vi "Autonomous.vi"   [LabVIEW 2019]
doc: "This VI starts when autonomous period begins, and will automatically be terminated when it ends. You can carry out timed or sensor driven operations directly to I/O or to subsystems without needing to return to the caller."
uses:
  <vilib>/Rock Robotics/WPI/Solenoid/WPI_SolenoidValue.ctl
  <vilib>/Rock Robotics/Network Tables/NT Read String.vi
  Framework/Robot Global Data.vi
types:
  T1 = typedef "WPI_SolenoidValue.ctl" = enum16{"Off", "On", "Forward", "Reverse"}
  T2 = typedef "Command Status Info.ctl" = cluster{"Name":string, "Status":T3, "notifier out":T4}
  T3 = typedef "Completion Status.ctl" = enum16{"Successful", "Aborted", "Incomplete"}
  T4 = typedef "Completion Notifier.ctl" = refnum<notifier>
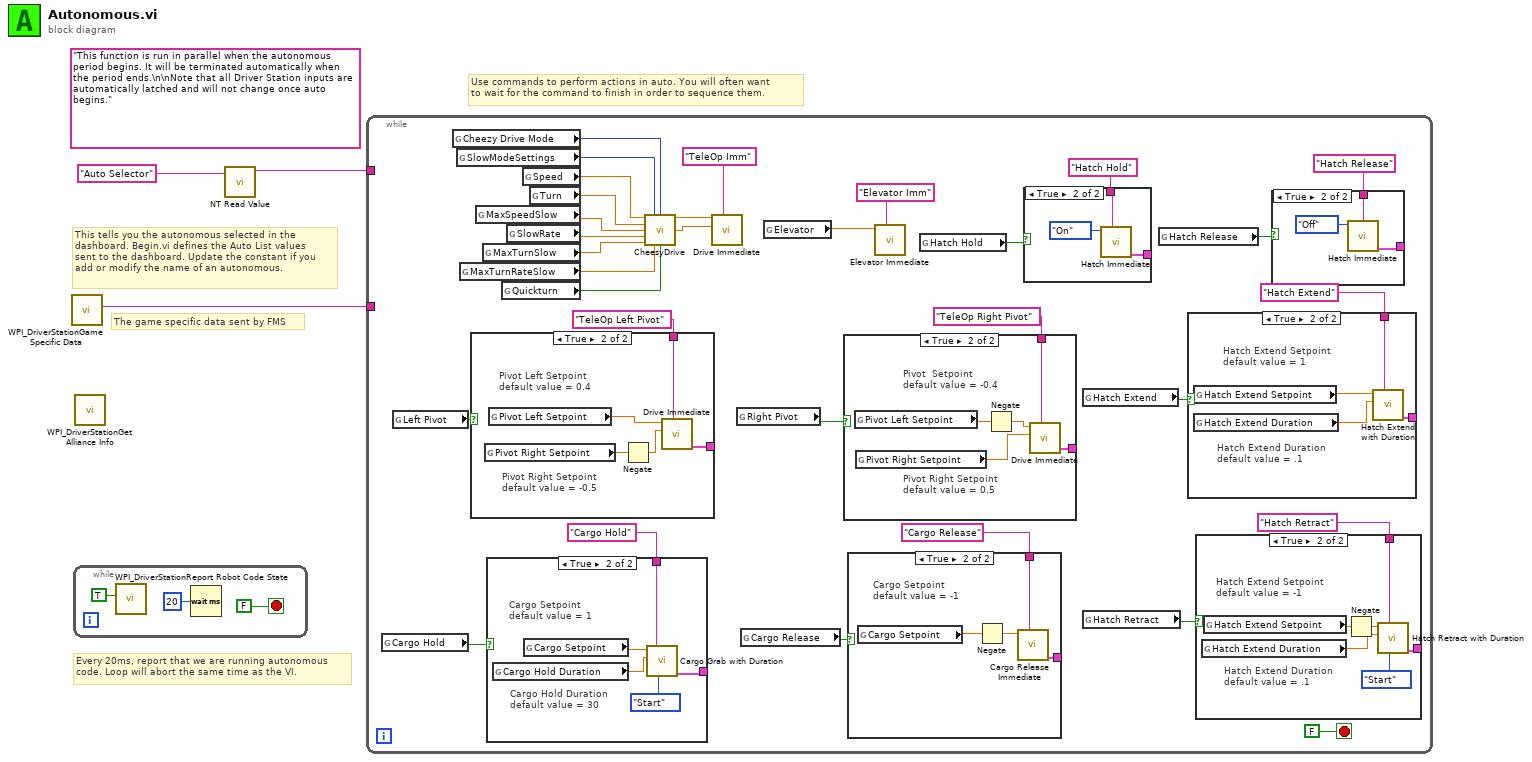
[diagram p0: block diagram]
diagram:
  (unwired) "This function is run in parallel when the autonomous period begins. It will be terminated automatically when the period ends.\n\nNote that all Driver Station inputs are automatically latched and will not change once auto begins."
  # "The game specific data sent by FMS"
  # "This tells you the autonomous selected in the \ndashboard. Begin.vi defines the Auto List values\nsent to the dashboard. Update the constant if you\nadd or modify the name of an autonomous."
  # "Every 20ms, report that we are running autonomous\ncode. Loop will abort the same time as the VI."
  # "Use commands to perform actions in auto. You will often want\nto wait for the command to finish in order to sequence them."
  n1 = call <vilib>:"WPI_DriverStationGame Specific Data.vi"() -> ("Game Specific Data"=w1:string)  [unwired: 11 in]
  n2 = while {
    stop <- FALSE stop-if-true
    n3 = call <vilib>:"WPI_DriverStationReport Robot Code State.vi"("Autonomous"=TRUE) -> ()  [unwired: 10 in, 1 out]
    n4 = Wait (ms)(milliseconds to wait=u32 20) -> ()  [unwired: 1 out]
  }
  n5 = call <vilib>:"WPI_DriverStationGet Alliance Info.vi"() -> ()  [unwired: 12 out]
  n6 = call-poly <vilib>:"NT Read Value.vi"("Name"="Auto Selector") -> ("String"=w2:string)  [unwired: 9 in, 1 out]
  n7 = while {
    tunnel: w2 -> [_]
    tunnel: w1 -> [_]
    stop <- FALSE stop-if-true
    n8 = global read "Robot Global Data.vi" "Cargo Hold"() -> (w17:bool)
    n9 = global read "Robot Global Data.vi" "Left Pivot"() -> (w33:bool)
    n10 = global read "Robot Global Data.vi" "Cheezy Drive Mode"() -> (w32:u32)
    n11 = global read "Robot Global Data.vi" "SlowModeSettings"() -> (w22:i32)
    n12 = global read "Robot Global Data.vi" "MaxTurnRateSlow"() -> (w24:dbl)
    n13 = case shown="True" w33 {
      tunnel: [_ w72] -> _
      tunnel: "TeleOp Left Pivot" ("Description") -> [_ w71]
      frame False {
      }
      frame True {
        # "Pivot Right Setpoint\ndefault value = -0.5"
        # "Pivot Left Setpoint\ndefault value = 0.4"
        n14 = global read "Robot Global Data.vi" "Pivot Right Setpoint"() -> (w69:dbl)
        n15 = global read "Robot Global Data.vi" "Pivot Left Setpoint"() -> (w70:dbl)
        n16 = Negate(x=w69) -> (-x=w68:dbl)
        n17 = call "Drive Immediate.vi"("Description"=w71, "Right Setpoint"=w68, "Left Setpoint"=w70) -> ("Command Info Out"=w72:T2)  [unwired: 8 in]
      }
    }
    n18 = global read "Robot Global Data.vi" "MaxSpeedSlow"() -> (w27:dbl)
    n19 = global read "Robot Global Data.vi" "MaxTurnSlow"() -> (w25:dbl)
    n20 = case shown="True" w17 {
      tunnel: [_ w62] -> _
      tunnel: "Cargo Hold" ("Description") -> [_ w61]
      frame False {
      }
      frame True {
        # "Cargo Hold Duration\ndefault value = 30"
        # "Cargo Setpoint\ndefault value = 1"
        n21 = global read "Robot Global Data.vi" "Cargo Hold Duration"() -> (w58:dbl)
        n22 = global read "Robot Global Data.vi" "Cargo Setpoint"() -> (w60:dbl)
        n23 = call "Cargo Grab with Duration.vi"("Synchronization"=enum16{"Start", "Wait"}."Start", "Description"=w61, "Duration (s)"=w58, "Setpoint"=w60) -> ("Command Info Out"=w62:T2)  [unwired: 7 in]
      }
    }
    n24 = global read "Robot Global Data.vi" "Quickturn"() -> (w23:bool)
    n25 = global read "Robot Global Data.vi" "SlowRate"() -> (w26:dbl)
    n26 = global read "Robot Global Data.vi" "Speed"() -> (w29:dbl)
    n27 = global read "Robot Global Data.vi" "Turn"() -> (w28:dbl)
    n28 = call "CheesyDrive.vi"("Throttle"=w29, "SlowModeSettings"=w22, "SlowMode"=w32, "Wheel"=w28, "MaxSpeedSlow"=w27, "SlowRate"=w26, "MaxTurnSlow"=w25, "MaxTurnRateSlow"=w24, "Quickturn"=w23) -> ("Left PWM"=w31:dbl, "Right PWM"=w30:dbl)  [unwired: 5 in]
    n29 = call "Drive Immediate.vi"("Description"="TeleOp Imm", "Right Setpoint"=w30, "Left Setpoint"=w31) -> ()  [unwired: 8 in, 1 out]
    n30 = global read "Robot Global Data.vi" "Right Pivot"() -> (w34:bool)
    n31 = global read "Robot Global Data.vi" "Cargo Release"() -> (w16:bool)
    n32 = global read "Robot Global Data.vi" "Elevator"() -> (w21:dbl)
    n33 = case shown="True" w34 {
      tunnel: [_ w67] -> _
      tunnel: "TeleOp Right Pivot" ("Description") -> [_ w66]
      frame False {
      }
      frame True {
        # "Pivot Right Setpoint\ndefault value = 0.5"
        # "Pivot  Setpoint\ndefault value = -0.4"
        n34 = global read "Robot Global Data.vi" "Pivot Left Setpoint"() -> (w64:dbl)
        n35 = global read "Robot Global Data.vi" "Pivot Right Setpoint"() -> (w65:dbl)
        n36 = Negate(x=w64) -> (-x=w63:dbl)
        n37 = call "Drive Immediate.vi"("Description"=w66, "Right Setpoint"=w65, "Left Setpoint"=w63) -> ("Command Info Out"=w67:T2)  [unwired: 8 in]
      }
    }
    n38 = case shown="True" w16 {
      tunnel: [_ w57] -> _
      tunnel: "Cargo Release" ("Description") -> [_ w56]
      frame False {
      }
      frame True {
        # "Cargo Setpoint\ndefault value = -1"
        n39 = global read "Robot Global Data.vi" "Cargo Setpoint"() -> (w55:dbl)
        n40 = Negate(x=w55) -> (-x=w54:dbl)
        n41 = call "Cargo Release Immediate.vi"("Description"=w56, "Setpoint"=w54) -> ("Command Info Out"=w57:T2)  [unwired: 9 in]
      }
    }
    n42 = call "Elevator Immediate.vi"("Description"="Elevator Imm", "Setpoint"=w21) -> ()  [unwired: 9 in, 1 out]
    n43 = global read "Robot Global Data.vi" "Hatch Hold"() -> (w12:bool)
    n44 = case shown="True" w12 {
      tunnel: "Hatch Hold" ("Description") -> [_ w53]
      tunnel: [_ w52] -> _
      frame False {
      }
      frame True {
        n45 = call "Hatch Immediate.vi"("Description"=w53, "Relay Value"=WPI_SolenoidValue."On" ("Hatch Action")) -> ("Command Info Out"=w52:T2)  [unwired: 9 in]
      }
    }
    n46 = global read "Robot Global Data.vi" "Hatch Extend"() -> (w9:bool)
    n47 = global read "Robot Global Data.vi" "Hatch Retract"() -> (w10:bool)
    n48 = global read "Robot Global Data.vi" "Hatch Release"() -> (w13:bool)
    n49 = case shown="True" w9 {
      tunnel: [_ w41] -> _
      tunnel: "Hatch Extend" ("Description") -> [_ w40]
      frame False {
      }
      frame True {
        # "Hatch Extend Duration\ndefault value = .1"
        # "Hatch Extend Setpoint\ndefault value = 1"
        n50 = global read "Robot Global Data.vi" "Hatch Extend Setpoint"() -> (w39:dbl)
        n51 = global read "Robot Global Data.vi" "Hatch Extend Duration"() -> (w38:dbl)
        n52 = call "Hatch Extend with Duration.vi"("Description"=w40, "Duration (s)"=w38, "Setpoint"=w39) -> ("Command Info Out"=w41:T2)  [unwired: 8 in]
      }
    }
    n53 = case shown="True" w10 {
      tunnel: [_ w47] -> _
      tunnel: "Hatch Retract" ("Description") -> [_ w46]
      frame False {
      }
      frame True {
        # "Hatch Extend Setpoint\ndefault value = -1"
        # "Hatch Extend Duration\ndefault value = .1"
        n54 = global read "Robot Global Data.vi" "Hatch Extend Duration"() -> (w43:dbl)
        n55 = global read "Robot Global Data.vi" "Hatch Extend Setpoint"() -> (w45:dbl)
        n56 = Negate(x=w45) -> (-x=w42:dbl)
        n57 = call "Hatch Retract with Duration.vi"("Synchronization"=enum16{"Start", "Wait"}."Start", "Description"=w46, "Duration (s)"=w43, "Setpoint"=w42) -> ("Command Info Out"=w47:T2)  [unwired: 7 in]
      }
    }
    n58 = case shown="True" w13 {
      tunnel: "Hatch Release" ("Description") -> [_ w50]
      tunnel: [_ w49] -> _
      frame False {
      }
      frame True {
        n59 = call "Hatch Immediate.vi"("Description"=w50, "Relay Value"=WPI_SolenoidValue."Off" ("Hatch Action")) -> ("Command Info Out"=w49:T2)  [unwired: 9 in]
      }
    }
  }
